vi "Komponenten Formeln Finden.vi"(10 "Komponenten Alt":T1 {"Komponente 5"."Komponente:" items=["NO (350,3000) LP 191C", "NO2 (150) LP 191C (1of2)", "NO2 (2000) LP 191C (2of2)", "N2O (300) LP 191C (1of2)", "NH3 (300) LP 191C (1of2)", "NH3 (900,3000) LP 191C (2of2)", "HNCO (400) 191C", "H2O% (30) LP 191C", "Formaldehyde (70,500) LP 191C", "CO2 low% (4) LP 191C (2of2)", "CO2% (20) LP 191C (1of2)", "CO (700) LP 191C (1of3)", "CO% (1) LP 191C (2of3)", "Propylene (1000) LP 191C", "Aromatic HC C7 (500) LP 191C", "Ethylene (1000) LP 191C", "CH4 (250) LP 191C (1of2)", "CH4 (5000) LP 191C (2of2)", "Ethane (1000) LP 191C", "Acetylene (1000) LP 191C", "HNO2 (20) 191C", "MeOH (1000) 191C", "CO% (10) LP 191C (3of3)", "Formic Acid (100) 191C", "SO2 (500) LP 191C", "Acetaldehyde (1000) LP 191C", "COS (100) LP 191C", "1,3 butadiene (100) LP 191C", "Oil as Octane (200) LP 191C", "N2O (1000) LP 191C (2of2)", "Propane (200) LP 191C", "NO2 autorange (2000)", "CO autorange (100000)", "CH4 autorange (5000)", "NH3 autorange (3000)", "Temp. Gascell", "Pressure Gascell", "sBeam@2500"]; "Komponente 5"."Konzentration IST" format="%#.4f"; "Komponente 5"."Genauigkeit" format="%#.1f"; "Komponente 4"."Komponente:" items=["NO (350,3000) LP 191C", "NO2 (150) LP 191C (1of2)", "NO2 (2000) LP 191C (2of2)", "N2O (300) LP 191C (1of2)", "NH3 (300) LP 191C (1of2)", "NH3 (900,3000) LP 191C (2of2)", "HNCO (400) 191C", "H2O% (30) LP 191C", "Formaldehyde (70,500) LP 191C", "CO2 low% (4) LP 191C (2of2)", "CO2% (20) LP 191C (1of2)", "CO (700) LP 191C (1of3)", "CO% (1) LP 191C (2of3)", "Propylene (1000) LP 191C", "Aromatic HC C7 (500) LP 191C", "Ethylene (1000) LP 191C", "CH4 (250) LP 191C (1of2)", "CH4 (5000) LP 191C (2of2)", "Ethane (1000) LP 191C", "Acetylene (1000) LP 191C", "HNO2 (20) 191C", "MeOH (1000) 191C", "CO% (10) LP 191C (3of3)", "Formic Acid (100) 191C", "SO2 (500) LP 191C", "Acetaldehyde (1000) LP 191C", "COS (100) LP 191C", "1,3 butadiene (100) LP 191C", "Oil as Octane (200) LP 191C", "N2O (1000) LP 191C (2of2)", "Propane (200) LP 191C", "NO2 autorange (2000)", "CO autorange (100000)", "CH4 autorange (5000)", "NH3 autorange (3000)", "Temp. Gascell", "Pressure Gascell", "sBeam@2500"]; "Komponente 4"."Konzentration IST" format="%#.4f"; "Komponente 4"."Genauigkeit" format="%#.1f"; "Komponente 3"."Komponente:" items=["NO (350,3000) LP 191C", "NO2 (150) LP 191C (1of2)", "NO2 (2000) LP 191C (2of2)", "N2O (300) LP 191C (1of2)", "NH3 (300) LP 191C (1of2)", "NH3 (900,3000) LP 191C (2of2)", "HNCO (400) 191C", "H2O% (30) LP 191C", "Formaldehyde (70,500) LP 191C", "CO2 low% (4) LP 191C (2of2)", "CO2% (20) LP 191C (1of2)", "CO (700) LP 191C (1of3)", "CO% (1) LP 191C (2of3)", "Propylene (1000) LP 191C", "Aromatic HC C7 (500) LP 191C", "Ethylene (1000) LP 191C", "CH4 (250) LP 191C (1of2)", "CH4 (5000) LP 191C (2of2)", "Ethane (1000) LP 191C", "Acetylene (1000) LP 191C", "HNO2 (20) 191C", "MeOH (1000) 191C", "CO% (10) LP 191C (3of3)", "Formic Acid (100) 191C", "SO2 (500) LP 191C", "Acetaldehyde (1000) LP 191C", "COS (100) LP 191C", "1,3 butadiene (100) LP 191C", "Oil as Octane (200) LP 191C", "N2O (1000) LP 191C (2of2)", "Propane (200) LP 191C", "NO2 autorange (2000)", "CO autorange (100000)", "CH4 autorange (5000)", "NH3 autorange (3000)", "Temp. Gascell", "Pressure Gascell", "sBeam@2500"]; "Komponente 3"."Konzentration IST" format="%#.4f"; "Komponente 3"."Genauigkeit" format="%#.1f"; "Komponente 2"."Komponente:" items=["NO (350,3000) LP 191C", "NO2 (150) LP 191C (1of2)", "NO2 (2000) LP 191C (2of2)", "N2O (300) LP 191C (1of2)", "NH3 (300) LP 191C (1of2)", "NH3 (900,3000) LP 191C (2of2)", "HNCO (400) 191C", "H2O% (30) LP 191C", "Formaldehyde (70,500) LP 191C", "CO2 low% (4) LP 191C (2of2)", "CO2% (20) LP 191C (1of2)", "CO (700) LP 191C (1of3)", "CO% (1) LP 191C (2of3)", "Propylene (1000) LP 191C", "Aromatic HC C7 (500) LP 191C", "Ethylene (1000) LP 191C", "CH4 (250) LP 191C (1of2)", "CH4 (5000) LP 191C (2of2)", "Ethane (1000) LP 191C", "Acetylene (1000) LP 191C", "HNO2 (20) 191C", "MeOH (1000) 191C", "CO% (10) LP 191C (3of3)", "Formic Acid (100) 191C", "SO2 (500) LP 191C", "Acetaldehyde (1000) LP 191C", "COS (100) LP 191C", "1,3 butadiene (100) LP 191C", "Oil as Octane (200) LP 191C", "N2O (1000) LP 191C (2of2)", "Propane (200) LP 191C", "NO2 autorange (2000)", "CO autorange (100000)", "CH4 autorange (5000)", "NH3 autorange (3000)", "Temp. Gascell", "Pressure Gascell", "sBeam@2500"]; "Komponente 2"."Konzentration IST" format="%#.4f"; "Komponente 2"."Genauigkeit" format="%#.1f"; "Komponente 1"."Komponente:" items=["NO (350,3000) LP 191C", "NO2 (150) LP 191C (1of2)", "NO2 (2000) LP 191C (2of2)", "N2O (300) LP 191C (1of2)", "NH3 (300) LP 191C (1of2)", "NH3 (900,3000) LP 191C (2of2)", "HNCO (400) 191C", "H2O% (30) LP 191C", "Formaldehyde (70,500) LP 191C", "CO2 low% (4) LP 191C (2of2)", "CO2% (20) LP 191C (1of2)", "CO (700) LP 191C (1of3)", "CO% (1) LP 191C (2of3)", "Propylene (1000) LP 191C", "Aromatic HC C7 (500) LP 191C", "Ethylene (1000) LP 191C", "CH4 (250) LP 191C (1of2)", "CH4 (5000) LP 191C (2of2)", "Ethane (1000) LP 191C", "Acetylene (1000) LP 191C", "HNO2 (20) 191C", "MeOH (1000) 191C", "CO% (10) LP 191C (3of3)", "Formic Acid (100) 191C", "SO2 (500) LP 191C", "Acetaldehyde (1000) LP 191C", "COS (100) LP 191C", "1,3 butadiene (100) LP 191C", "Oil as Octane (200) LP 191C", "N2O (1000) LP 191C (2of2)", "Propane (200) LP 191C", "NO2 autorange (2000)", "CO autorange (100000)", "CH4 autorange (5000)", "NH3 autorange (3000)", "Temp. Gascell", "Pressure Gascell", "sBeam@2500"]; "Komponente 1"."Konzentration IST" format="%#.4f"; "Komponente 1"."Genauigkeit" format="%#.1f"}, 11 "Komponenten (Eingang)":T1 {"Komponente 5"."Komponente:" items=["NO (350,3000) LP 191C", "NO2 (150) LP 191C (1of2)", "NO2 (2000) LP 191C (2of2)", "N2O (300) LP 191C (1of2)", "NH3 (300) LP 191C (1of2)", "NH3 (900,3000) LP 191C (2of2)", "HNCO (400) 191C", "H2O% (30) LP 191C", "Formaldehyde (70,500) LP 191C", "CO2 low% (4) LP 191C (2of2)", "CO2% (20) LP 191C (1of2)", "CO (700) LP 191C (1of3)", "CO% (1) LP 191C (2of3)", "Propylene (1000) LP 191C", "Aromatic HC C7 (500) LP 191C", "Ethylene (1000) LP 191C", "CH4 (250) LP 191C (1of2)", "CH4 (5000) LP 191C (2of2)", "Ethane (1000) LP 191C", "Acetylene (1000) LP 191C", "HNO2 (20) 191C", "MeOH (1000) 191C", "CO% (10) LP 191C (3of3)", "Formic Acid (100) 191C", "SO2 (500) LP 191C", "Acetaldehyde (1000) LP 191C", "COS (100) LP 191C", "1,3 butadiene (100) LP 191C", "Oil as Octane (200) LP 191C", "N2O (1000) LP 191C (2of2)", "Propane (200) LP 191C", "NO2 autorange (2000)", "CO autorange (100000)", "CH4 autorange (5000)", "NH3 autorange (3000)", "Temp. Gascell", "Pressure Gascell", "sBeam@2500"]; "Komponente 5"."Konzentration IST" format="%#.4f"; "Komponente 5"."Genauigkeit" format="%#.1f"; "Komponente 4"."Komponente:" items=["NO (350,3000) LP 191C", "NO2 (150) LP 191C (1of2)", "NO2 (2000) LP 191C (2of2)", "N2O (300) LP 191C (1of2)", "NH3 (300) LP 191C (1of2)", "NH3 (900,3000) LP 191C (2of2)", "HNCO (400) 191C", "H2O% (30) LP 191C", "Formaldehyde (70,500) LP 191C", "CO2 low% (4) LP 191C (2of2)", "CO2% (20) LP 191C (1of2)", "CO (700) LP 191C (1of3)", "CO% (1) LP 191C (2of3)", "Propylene (1000) LP 191C", "Aromatic HC C7 (500) LP 191C", "Ethylene (1000) LP 191C", "CH4 (250) LP 191C (1of2)", "CH4 (5000) LP 191C (2of2)", "Ethane (1000) LP 191C", "Acetylene (1000) LP 191C", "HNO2 (20) 191C", "MeOH (1000) 191C", "CO% (10) LP 191C (3of3)", "Formic Acid (100) 191C", "SO2 (500) LP 191C", "Acetaldehyde (1000) LP 191C", "COS (100) LP 191C", "1,3 butadiene (100) LP 191C", "Oil as Octane (200) LP 191C", "N2O (1000) LP 191C (2of2)", "Propane (200) LP 191C", "NO2 autorange (2000)", "CO autorange (100000)", "CH4 autorange (5000)", "NH3 autorange (3000)", "Temp. Gascell", "Pressure Gascell", "sBeam@2500"]; "Komponente 4"."Konzentration IST" format="%#.4f"; "Komponente 4"."Genauigkeit" format="%#.1f"; "Komponente 3"."Komponente:" items=["NO (350,3000) LP 191C", "NO2 (150) LP 191C (1of2)", "NO2 (2000) LP 191C (2of2)", "N2O (300) LP 191C (1of2)", "NH3 (300) LP 191C (1of2)", "NH3 (900,3000) LP 191C (2of2)", "HNCO (400) 191C", "H2O% (30) LP 191C", "Formaldehyde (70,500) LP 191C", "CO2 low% (4) LP 191C (2of2)", "CO2% (20) LP 191C (1of2)", "CO (700) LP 191C (1of3)", "CO% (1) LP 191C (2of3)", "Propylene (1000) LP 191C", "Aromatic HC C7 (500) LP 191C", "Ethylene (1000) LP 191C", "CH4 (250) LP 191C (1of2)", "CH4 (5000) LP 191C (2of2)", "Ethane (1000) LP 191C", "Acetylene (1000) LP 191C", "HNO2 (20) 191C", "MeOH (1000) 191C", "CO% (10) LP 191C (3of3)", "Formic Acid (100) 191C", "SO2 (500) LP 191C", "Acetaldehyde (1000) LP 191C", "COS (100) LP 191C", "1,3 butadiene (100) LP 191C", "Oil as Octane (200) LP 191C", "N2O (1000) LP 191C (2of2)", "Propane (200) LP 191C", "NO2 autorange (2000)", "CO autorange (100000)", "CH4 autorange (5000)", "NH3 autorange (3000)", "Temp. Gascell", "Pressure Gascell", "sBeam@2500"]; "Komponente 3"."Konzentration IST" format="%#.4f"; "Komponente 3"."Genauigkeit" format="%#.1f"; "Komponente 2"."Komponente:" items=["NO (350,3000) LP 191C", "NO2 (150) LP 191C (1of2)", "NO2 (2000) LP 191C (2of2)", "N2O (300) LP 191C (1of2)", "NH3 (300) LP 191C (1of2)", "NH3 (900,3000) LP 191C (2of2)", "HNCO (400) 191C", "H2O% (30) LP 191C", "Formaldehyde (70,500) LP 191C", "CO2 low% (4) LP 191C (2of2)", "CO2% (20) LP 191C (1of2)", "CO (700) LP 191C (1of3)", "CO% (1) LP 191C (2of3)", "Propylene (1000) LP 191C", "Aromatic HC C7 (500) LP 191C", "Ethylene (1000) LP 191C", "CH4 (250) LP 191C (1of2)", "CH4 (5000) LP 191C (2of2)", "Ethane (1000) LP 191C", "Acetylene (1000) LP 191C", "HNO2 (20) 191C", "MeOH (1000) 191C", "CO% (10) LP 191C (3of3)", "Formic Acid (100) 191C", "SO2 (500) LP 191C", "Acetaldehyde (1000) LP 191C", "COS (100) LP 191C", "1,3 butadiene (100) LP 191C", "Oil as Octane (200) LP 191C", "N2O (1000) LP 191C (2of2)", "Propane (200) LP 191C", "NO2 autorange (2000)", "CO autorange (100000)", "CH4 autorange (5000)", "NH3 autorange (3000)", "Temp. Gascell", "Pressure Gascell", "sBeam@2500"]; "Komponente 2"."Konzentration IST" format="%#.4f"; "Komponente 2"."Genauigkeit" format="%#.1f"; "Komponente 1"."Komponente:" items=["NO (350,3000) LP 191C", "NO2 (150) LP 191C (1of2)", "NO2 (2000) LP 191C (2of2)", "N2O (300) LP 191C (1of2)", "NH3 (300) LP 191C (1of2)", "NH3 (900,3000) LP 191C (2of2)", "HNCO (400) 191C", "H2O% (30) LP 191C", "Formaldehyde (70,500) LP 191C", "CO2 low% (4) LP 191C (2of2)", "CO2% (20) LP 191C (1of2)", "CO (700) LP 191C (1of3)", "CO% (1) LP 191C (2of3)", "Propylene (1000) LP 191C", "Aromatic HC C7 (500) LP 191C", "Ethylene (1000) LP 191C", "CH4 (250) LP 191C (1of2)", "CH4 (5000) LP 191C (2of2)", "Ethane (1000) LP 191C", "Acetylene (1000) LP 191C", "HNO2 (20) 191C", "MeOH (1000) 191C", "CO% (10) LP 191C (3of3)", "Formic Acid (100) 191C", "SO2 (500) LP 191C", "Acetaldehyde (1000) LP 191C", "COS (100) LP 191C", "1,3 butadiene (100) LP 191C", "Oil as Octane (200) LP 191C", "N2O (1000) LP 191C (2of2)", "Propane (200) LP 191C", "NO2 autorange (2000)", "CO autorange (100000)", "CH4 autorange (5000)", "NH3 autorange (3000)", "Temp. Gascell", "Pressure Gascell", "sBeam@2500"]; "Komponente 1"."Konzentration IST" format="%#.4f"; "Komponente 1"."Genauigkeit" format="%#.1f"}) -> (3 "Komponenten (Ausgang)":T1 {"Komponente 5"."Komponente:" items=["NO (350,3000) LP 191C", "NO2 (150) LP 191C (1of2)", "NO2 (2000) LP 191C (2of2)", "N2O (300) LP 191C (1of2)", "NH3 (300) LP 191C (1of2)", "NH3 (900,3000) LP 191C (2of2)", "HNCO (400) 191C", "H2O% (30) LP 191C", "Formaldehyde (70,500) LP 191C", "CO2 low% (4) LP 191C (2of2)", "CO2% (20) LP 191C (1of2)", "CO (700) LP 191C (1of3)", "CO% (1) LP 191C (2of3)", "Propylene (1000) LP 191C", "Aromatic HC C7 (500) LP 191C", "Ethylene (1000) LP 191C", "CH4 (250) LP 191C (1of2)", "CH4 (5000) LP 191C (2of2)", "Ethane (1000) LP 191C", "Acetylene (1000) LP 191C", "HNO2 (20) 191C", "MeOH (1000) 191C", "CO% (10) LP 191C (3of3)", "Formic Acid (100) 191C", "SO2 (500) LP 191C", "Acetaldehyde (1000) LP 191C", "COS (100) LP 191C", "1,3 butadiene (100) LP 191C", "Oil as Octane (200) LP 191C", "N2O (1000) LP 191C (2of2)", "Propane (200) LP 191C", "NO2 autorange (2000)", "CO autorange (100000)", "CH4 autorange (5000)", "NH3 autorange (3000)", "Temp. Gascell", "Pressure Gascell", "sBeam@2500"]; "Komponente 5"."Konzentration IST" format="%#.4f"; "Komponente 5"."Genauigkeit" format="%#.1f"; "Komponente 4"."Komponente:" items=["NO (350,3000) LP 191C", "NO2 (150) LP 191C (1of2)", "NO2 (2000) LP 191C (2of2)", "N2O (300) LP 191C (1of2)", "NH3 (300) LP 191C (1of2)", "NH3 (900,3000) LP 191C (2of2)", "HNCO (400) 191C", "H2O% (30) LP 191C", "Formaldehyde (70,500) LP 191C", "CO2 low% (4) LP 191C (2of2)", "CO2% (20) LP 191C (1of2)", "CO (700) LP 191C (1of3)", "CO% (1) LP 191C (2of3)", "Propylene (1000) LP 191C", "Aromatic HC C7 (500) LP 191C", "Ethylene (1000) LP 191C", "CH4 (250) LP 191C (1of2)", "CH4 (5000) LP 191C (2of2)", "Ethane (1000) LP 191C", "Acetylene (1000) LP 191C", "HNO2 (20) 191C", "MeOH (1000) 191C", "CO% (10) LP 191C (3of3)", "Formic Acid (100) 191C", "SO2 (500) LP 191C", "Acetaldehyde (1000) LP 191C", "COS (100) LP 191C", "1,3 butadiene (100) LP 191C", "Oil as Octane (200) LP 191C", "N2O (1000) LP 191C (2of2)", "Propane (200) LP 191C", "NO2 autorange (2000)", "CO autorange (100000)", "CH4 autorange (5000)", "NH3 autorange (3000)", "Temp. Gascell", "Pressure Gascell", "sBeam@2500"]; "Komponente 4"."Konzentration IST" format="%#.4f"; "Komponente 4"."Genauigkeit" format="%#.1f"; "Komponente 3"."Komponente:" items=["NO (350,3000) LP 191C", "NO2 (150) LP 191C (1of2)", "NO2 (2000) LP 191C (2of2)", "N2O (300) LP 191C (1of2)", "NH3 (300) LP 191C (1of2)", "NH3 (900,3000) LP 191C (2of2)", "HNCO (400) 191C", "H2O% (30) LP 191C", "Formaldehyde (70,500) LP 191C", "CO2 low% (4) LP 191C (2of2)", "CO2% (20) LP 191C (1of2)", "CO (700) LP 191C (1of3)", "CO% (1) LP 191C (2of3)", "Propylene (1000) LP 191C", "Aromatic HC C7 (500) LP 191C", "Ethylene (1000) LP 191C", "CH4 (250) LP 191C (1of2)", "CH4 (5000) LP 191C (2of2)", "Ethane (1000) LP 191C", "Acetylene (1000) LP 191C", "HNO2 (20) 191C", "MeOH (1000) 191C", "CO% (10) LP 191C (3of3)", "Formic Acid (100) 191C", "SO2 (500) LP 191C", "Acetaldehyde (1000) LP 191C", "COS (100) LP 191C", "1,3 butadiene (100) LP 191C", "Oil as Octane (200) LP 191C", "N2O (1000) LP 191C (2of2)", "Propane (200) LP 191C", "NO2 autorange (2000)", "CO autorange (100000)", "CH4 autorange (5000)", "NH3 autorange (3000)", "Temp. Gascell", "Pressure Gascell", "sBeam@2500"]; "Komponente 3"."Konzentration IST" format="%#.4f"; "Komponente 3"."Genauigkeit" format="%#.1f"; "Komponente 2"."Komponente:" items=["NO (350,3000) LP 191C", "NO2 (150) LP 191C (1of2)", "NO2 (2000) LP 191C (2of2)", "N2O (300) LP 191C (1of2)", "NH3 (300) LP 191C (1of2)", "NH3 (900,3000) LP 191C (2of2)", "HNCO (400) 191C", "H2O% (30) LP 191C", "Formaldehyde (70,500) LP 191C", "CO2 low% (4) LP 191C (2of2)", "CO2% (20) LP 191C (1of2)", "CO (700) LP 191C (1of3)", "CO% (1) LP 191C (2of3)", "Propylene (1000) LP 191C", "Aromatic HC C7 (500) LP 191C", "Ethylene (1000) LP 191C", "CH4 (250) LP 191C (1of2)", "CH4 (5000) LP 191C (2of2)", "Ethane (1000) LP 191C", "Acetylene (1000) LP 191C", "HNO2 (20) 191C", "MeOH (1000) 191C", "CO% (10) LP 191C (3of3)", "Formic Acid (100) 191C", "SO2 (500) LP 191C", "Acetaldehyde (1000) LP 191C", "COS (100) LP 191C", "1,3 butadiene (100) LP 191C", "Oil as Octane (200) LP 191C", "N2O (1000) LP 191C (2of2)", "Propane (200) LP 191C", "NO2 autorange (2000)", "CO autorange (100000)", "CH4 autorange (5000)", "NH3 autorange (3000)", "Temp. Gascell", "Pressure Gascell", "sBeam@2500"]; "Komponente 2"."Konzentration IST" format="%#.4f"; "Komponente 2"."Genauigkeit" format="%#.1f"; "Komponente 1"."Komponente:" items=["NO (350,3000) LP 191C", "NO2 (150) LP 191C (1of2)", "NO2 (2000) LP 191C (2of2)", "N2O (300) LP 191C (1of2)", "NH3 (300) LP 191C (1of2)", "NH3 (900,3000) LP 191C (2of2)", "HNCO (400) 191C", "H2O% (30) LP 191C", "Formaldehyde (70,500) LP 191C", "CO2 low% (4) LP 191C (2of2)", "CO2% (20) LP 191C (1of2)", "CO (700) LP 191C (1of3)", "CO% (1) LP 191C (2of3)", "Propylene (1000) LP 191C", "Aromatic HC C7 (500) LP 191C", "Ethylene (1000) LP 191C", "CH4 (250) LP 191C (1of2)", "CH4 (5000) LP 191C (2of2)", "Ethane (1000) LP 191C", "Acetylene (1000) LP 191C", "HNO2 (20) 191C", "MeOH (1000) 191C", "CO% (10) LP 191C (3of3)", "Formic Acid (100) 191C", "SO2 (500) LP 191C", "Acetaldehyde (1000) LP 191C", "COS (100) LP 191C", "1,3 butadiene (100) LP 191C", "Oil as Octane (200) LP 191C", "N2O (1000) LP 191C (2of2)", "Propane (200) LP 191C", "NO2 autorange (2000)", "CO autorange (100000)", "CH4 autorange (5000)", "NH3 autorange (3000)", "Temp. Gascell", "Pressure Gascell", "sBeam@2500"]; "Komponente 1"."Konzentration IST" format="%#.4f"; "Komponente 1"."Genauigkeit" format="%#.1f"})   [LabVIEW 2020, in "Linearisierung v2.lvlib" / "SpanEinstellungen.lvlib"]
uses:
  SpanEinstellungen.lvlib
  Komponentencluster mit Formel.ctl
  Komponentenauswahl mit Formel.ctl
  Visualisierungs Elemente/String - Eingabefeld.ctl
  Einheit.ctl
  Gasteiler/Aktion FGV Gasteilerliste laden.ctl
  <vilib>/regexp/Match Regular Expression.xnode
  Gasteiler/Gasteiler.lvlib
panel:
  # "Komponente"
  # "Formel"
  # "Konzentration"
  # "Einheit"
  # "Genauigkeit [%]"
  # "Komponente"
  # "Formel"
  # "Konzentration"
  # "Einheit"
  # "Genauigkeit [%]"
  # "Komponente"
  # "Formel"
  # "Konzentration"
  # "Einheit"
  # "Genauigkeit [%]"
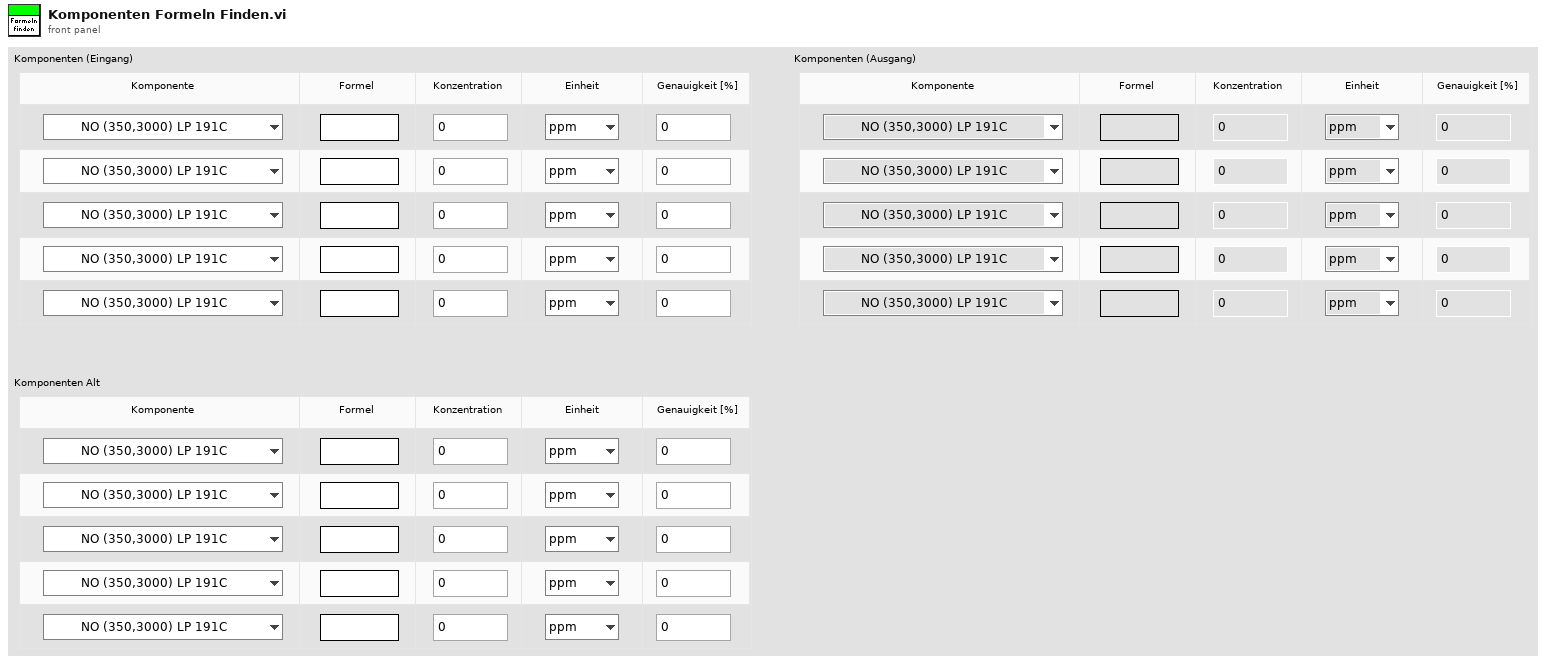
[diagram p1: front panel]
types:
  T1 = typedef "Linearisierung v2.lvlib/SpanEinstellungen.lvlib/Komponentencluster mit Formel.ctl" = cluster{"Komponente 1":T2, "Komponente 2":T2, "Komponente 3":T2, "Komponente 4":T2, "Komponente 5":T2}
  T2 = typedef "Linearisierung v2.lvlib/SpanEinstellungen.lvlib/Komponentenauswahl mit Formel.ctl" = cluster{"Komponente:":u16, "Summenformel":T3, "Konzentration IST":dbl, "Einheit":T4, "Genauigkeit":dbl}
  T3 = typedef "String - Eingabefeld.ctl" = string
  T4 = typedef "Linearisierung v2.lvlib/SpanEinstellungen.lvlib/Einheit.ctl" = enum16{"ppm", "%"}
  T5 = typedef "Linearisierung v2.lvlib/Gasteiler.lvlib/Aktion FGV Gasteilerliste laden.ctl" = enum16{"lesen", "laden", "speichern", "Liste erstellen", "Formel ändern", "Gas vereinzeln"}
  T6 = typedef "String - Ausgabefeld.ctl" = string
  T7 = cluster{"[0]":T2, "[1]":T2, "[2]":T2, "[3]":T2, "[4]":T2}
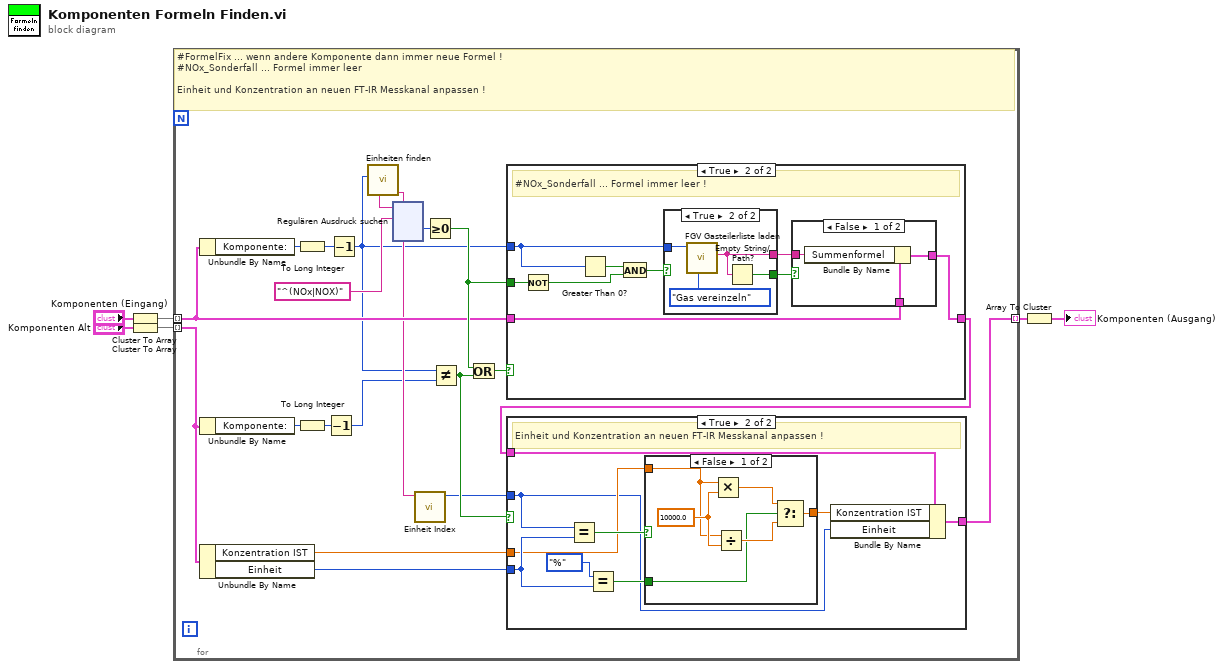
[diagram p0: block diagram]
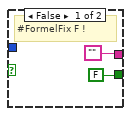
[diagram p5: hidden frame]
diagram:
  n1 = Cluster To Array(cluster="Komponenten (Eingang)") -> (array=w4:T2[])
  n2 = Cluster To Array(cluster="Komponenten Alt") -> (array=w3:T2[])
  n3 = for {
    tunnel: w3 -> [w18] mode=indexing
    tunnel: w4 -> [w15] mode=indexing
    tunnel: [w13] -> w2 mode=indexing
    # "#FormelFix ... wenn andere Komponente dann immer neue Formel !\n#NOx_Sonderfall ... Formel immer leer \n\nEinheit und Konzentration an neuen FT-IR Messkanal anpassen !"
    n4 = Unbundle By Name(w15) -> ("Komponente:"=w25:u16)
    n5 = Unbundle By Name(w18) -> ("Komponente:"=w26:u16)
    n6 = Unbundle By Name(w18) -> ("Konzentration IST"=w17:dbl, "Einheit"=w16:T4)
    n7 = To Long Integer(number=w25) -> (32bit integer=w10:i32)
    n8 = To Long Integer(number=w26) -> (32bit integer=w9:i32)
    n9 = Decrement(x=w9) -> (x-1=w7:i32)
    n10 = Decrement(x=w10) -> (x-1=w8:i32)
    n11 = call "Einheiten finden.vi"("Komponente"=w8) -> ("Einheit in String"=w12:string, "Komponenten Name"=w21:T6)  [unwired: 6 in, 3 out]
    n12 = xnode "Regulären Ausdruck suchen"("Eingangs-String"=w21, "Regulärer Ausdruck"="^(NOx|NOX)") -> ("Offset nach Übereinstimmung"=w20:i32)  [unwired: 4 in, 4 out]
    n13 = call "Einheit Index.vi"("Einheit in String"=w12) -> ("Elementindex"=w11:i32)  [unwired: 10 in]
    n14 = Greater Or Equal To 0?(x=w20) -> (x >= 0?=w22:bool)
    n15 = Not Equal?(x=w8, y=w7) -> (x != y?=w19:bool)
    n16 = Or(x=w22, y=w19) -> (x .or. y?=w23:bool)
    n17 = case shown="True" w23 {
      tunnel: w15 -> [w158 w167]
      tunnel: [w158 w166] -> w14
      tunnel: w8 -> [_ w163]
      tunnel: w22 -> [_ w160]
      frame False {
      }
      frame True {
        # "#NOx_Sonderfall ... Formel immer leer !"
        n18 = Not(x=w160) -> (.not. x?=w159:bool)
        n19 = Greater Than 0?(x=w163) -> (x > 0?=w162:bool)
        n20 = And(x=w162, y=w159) -> (x .and. y?=w161:bool)
        n21 = case shown="True" w161 {
          tunnel: w163 -> [_ w172]
          tunnel: ["" w171] -> w165
          tunnel: [FALSE w170] -> w164
          frame False {
            # "#FormelFix F !"
          }
          frame True {
            n22 = call "FGV Gasteilerliste laden.vi"("Aktion"=Aktion_FGV_Gasteilerliste_laden."Gas vereinzeln", "Gasindex"=w172) -> ("Formel"=w171:string)  [unwired: 7 in, 2 out]
            n23 = Empty String/Path?(string/path=w171) -> (empty?=w170:bool)
          }
        }
        n24 = case shown="False" w164 {
          tunnel: w167 -> [w176 w177]
          tunnel: [w175 w177] -> w166
          tunnel: w165 -> [w174 _]
          frame False {
            n25 = Bundle By Name(cluster=w176, "Summenformel"=w174) -> (w175:T2)
          }
          frame True {
          }
        }
      }
    }
    n26 = case shown="True" w19 {
      tunnel: w11 -> [_ w29]
      tunnel: w17 -> [_ w33]
      tunnel: w16 -> [_ w34]
      tunnel: w14 -> [w27 w31]
      tunnel: [w27 w28] -> w13
      frame False {
      }
      frame True {
        # "Einheit und Konzentration an neuen FT-IR Messkanal anpassen !"
        n27 = Equal?(x=w29, y=w34) -> (x = y?=w36:bool)
        n28 = Equal?(x=enum16{"ppm", "%"}."%" ("Einheit"), y=w34) -> (x = y?=w32:bool)
        n29 = case shown="False" w36 {
          tunnel: w33 -> [w40 w43]
          tunnel: [w38 w43] -> w30
          tunnel: w32 -> [w37 _]
          frame False {
            w41 = 10000.0 ("t")
            n30 = Multiply(x=w40, y=w41) -> (x*y=w42:dbl)
            n31 = Divide(x=w40, y=w41) -> (x/y=w39:dbl)
            n32 = Select(t=w42, s=w37, f=w39) -> (s? t:f=w38:dbl)
          }
          frame True {
          }
        }
        n33 = Bundle By Name(cluster=w31, "Konzentration IST"=w30, "Einheit"=w29) -> (w28:T2)
      }
    }
  }
  n34 = Array To Cluster(array=w2) -> (cluster=→"Komponenten (Ausgang)":T7)
